vi "MyFPGA Check DI IRQ.vi"(4 "Debounce Ticks":u16=5, 6 "Count":u32, 8 "On Falling Edge?":bool, 9 "On Rising Edge?":bool, 10 "Enable Interrupt?":bool, 11 "Digital In":bool) -> (3 "Trigger?":bool)   [LabVIEW 2019]
doc: "This VI checks if the digital input interrupt is triggered under the specified condition."
panel:
  # "This VI checks if the digital input interrupt is triggered under the specified condition."
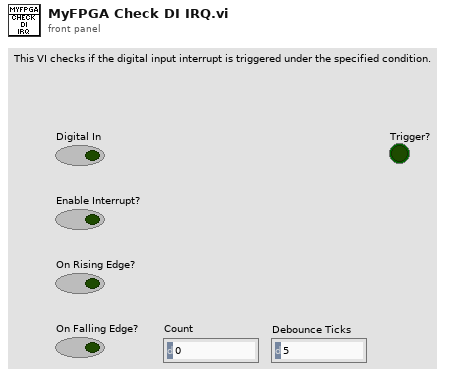
[diagram p1: front panel]
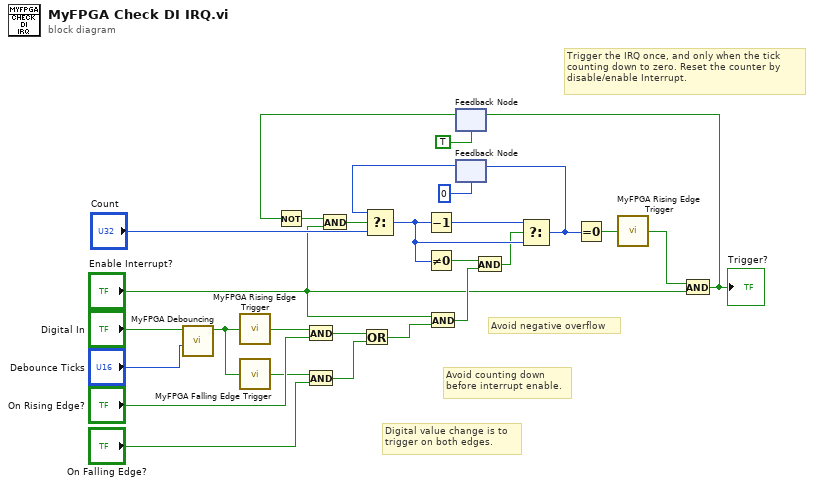
[diagram p0: block diagram]
diagram:
  # "Avoid counting down \nbefore interrupt enable."
  # "Trigger the IRQ once, and only when the tick \ncounting down to zero. Reset the counter by \ndisable/enable Interrupt."
  # "Avoid negative overflow"
  # "Digital value change is to \ntrigger on both edges."
  n1 = call "MyFPGA Debouncing.vi"("Debounce Ticks"="Debounce Ticks", "Input Signal"="Digital In") -> ("Debounced Signal"=w2:bool)  [unwired: 9 in]
  n2 = call "MyFPGA Rising Edge Trigger.vi"("Signal"=w2) -> ("Trigger?"=w25:bool)
  n3 = call "MyFPGA Falling Edge Trigger.vi"("Signal"=w2) -> ("Trigger?"=w24:bool)
  n4 = And(x=w25, y="On Rising Edge?") -> (x .and. y?=w23:bool)
  n5 = And(x=w24, y="On Falling Edge?") -> (x .and. y?=w22:bool)
  n6 = Or(x=w23, y=w22) -> (x .or. y?=w16:bool)
  n7 = And(x="Enable Interrupt?", y=w16) -> (x .and. y?=w13:bool)
  n8 = feedback #1(TRUE) -> (w5:bool)
  n9 = Not(x=w5) -> (.not. x?=w8:bool)
  n10 = And(x=w8, y="Enable Interrupt?") -> (x .and. y?=w6:bool)
  n11 = feedback #2(u32 0 ("Count")) -> (w18:u32)
  n12 = Select(t=w18, s=w6, f="Count") -> (s? t:f=w14:u32)
  n13 = Decrement(x=w14) -> (x-1=w15:u32)
  n14 = Not Equal To 0?(x=w14) -> (x != 0?=w12:bool)
  n15 = And(x=w12, y=w13) -> (x .and. y?=w11:bool)
  n16 = Select(t=w15, s=w11, f=w14) -> (s? t:f=w20:u32)
  n17 = feedback-in #2(w20) -> ()
  n18 = Equal To 0?(x=w20) -> (x = 0?=w19:bool)
  n19 = call "MyFPGA Rising Edge Trigger.vi"("Signal"=w19) -> ("Trigger?"=w10:bool)
  n20 = And(x=w10, y="Enable Interrupt?") -> (x .and. y?=w9:bool)
  "Trigger?" <- w9
  n21 = feedback-in #1(w9) -> ()
